vi "FGEN Configure Standard Waveform.vi"(4 "DC Offset (V)":dbl(knob) min=-6.0 max=6.0 scale=-6.0..6.0 scale format="%_1p", 6 "Start Phase":dbl, 7 "Standard Waveform":u16(slide) scale=0.0..6.0, 8 "error in (no error)":errorcluster, 9 "Amplitude (Vp-p)":dbl(knob)=1.0 min=0.0 max=12.0 scale=0.0..12.0 scale format="%.1f", 10 "Frequency (Hz)":dbl(knob)=1000000.0 min=9000.0 max=100000000.0 scale=0.0..100000000.0 scale format="%_1p", 11 "Function Generator in":refnum<class "Function Generator.lvclass">) -> (0 "error out":errorcluster, 3 "Function Generator out":refnum<class "Function Generator.lvclass">)   [LabVIEW 2023, in "HardwareAbstractionLayer_LVOOP.lvlib" / "Function Generator.lvclass"]
uses:
  Function Generator.lvclass
  Function Generator.lvclass/Function Generator.ctl
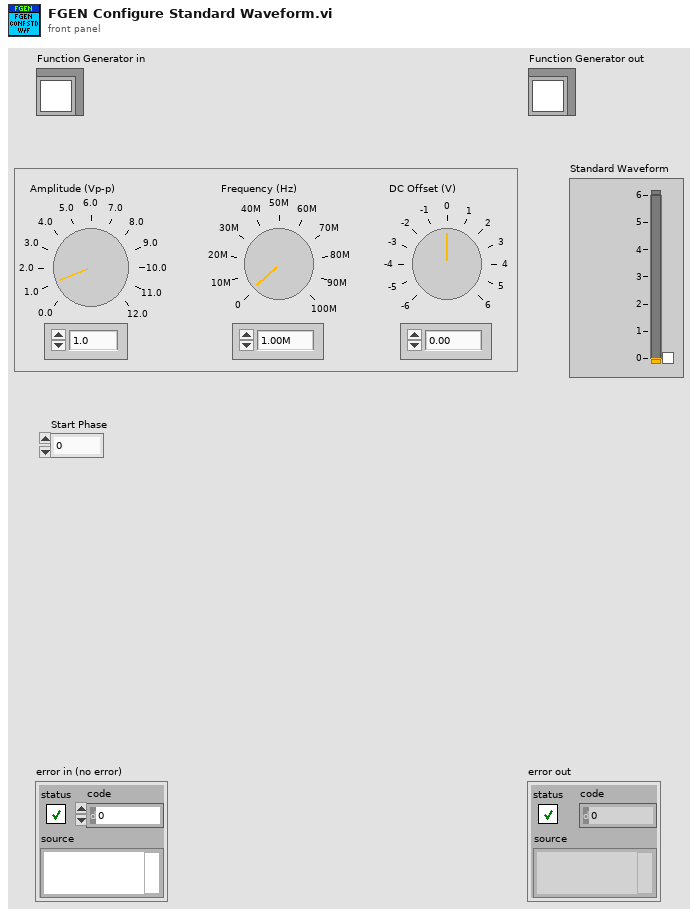
[diagram p1: front panel]
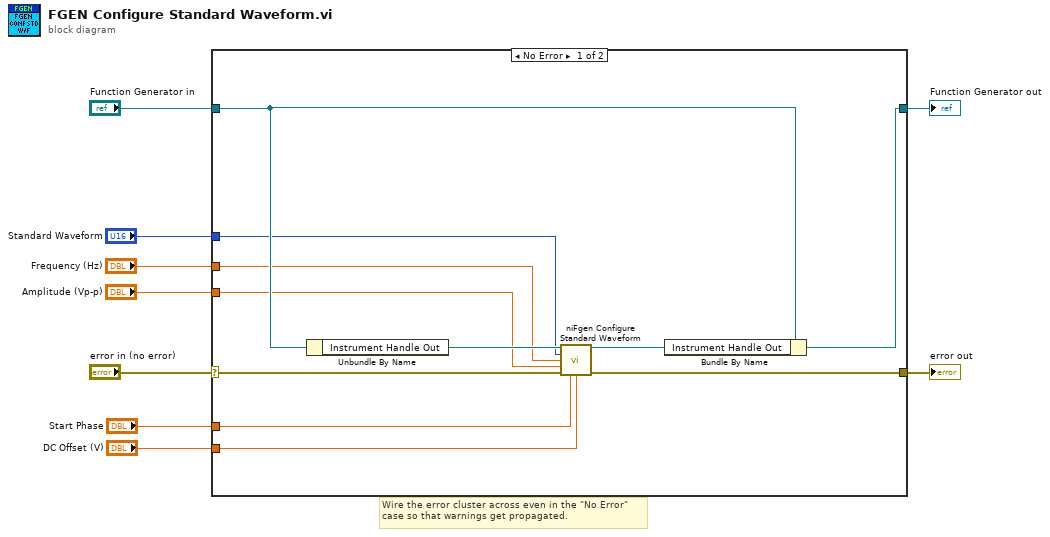
[diagram p0: block diagram]
diagram:
  # "Wire the error cluster across even in the \"No Error\"\ncase so that warnings get propagated."
  n1 = case shown="No Error" "error in (no error)" {
    selector: "error in (no error)" -> [w20 w22]
    tunnel: [w19 w22] -> w8
    tunnel: [w16 w21] -> w6
    tunnel: "Function Generator in" -> [w17 w21]
    tunnel: "Frequency (Hz)" -> [w14 _]
    tunnel: "Amplitude (Vp-p)" -> [w13 _]
    tunnel: "DC Offset (V)" -> [w12 _]
    tunnel: "Start Phase" -> [w11 _]
    tunnel: "Standard Waveform" -> [w10 _]
    frame No Error {
      n2 = Unbundle By Name(w17) -> ("Instrument Handle Out"=w18:refnum<k15>)
      n3 = call <instrlib>:"niFgen Configure Standard Waveform.vi"("Instrument Handle"=w18, "Waveform"=w10, "Frequency"=w14, "Amplitude"=w13, "error in (no error)"=w20, "Start Phase"=w11, "DC Offset"=w12) -> ("Instrument Handle Out"=w15:refnum<k15>, "error out"=w19:errorcluster)  [unwired: 7 in]
      n4 = Bundle By Name(cluster=w17, "Instrument Handle Out"=w15) -> (w16:refnum<class "Function Generator.lvclass">)
    }
    frame Error {
    }
  }
  "error out" <- w8
  "Function Generator out" <- w6
